vi "security_encrypt.vi"(3 "FORMULA":string, 4 "METHOD":u16(ring) items=["#0_none", "#1_hexa", "#2_hexa_scrambled"], 6 "RAW DATA":string) -> (0 "ENCRYPTED DATA":string)   [LabVIEW 2018, in "db_lib R3.lvlib"]
uses:
  db_lib R3.lvlib
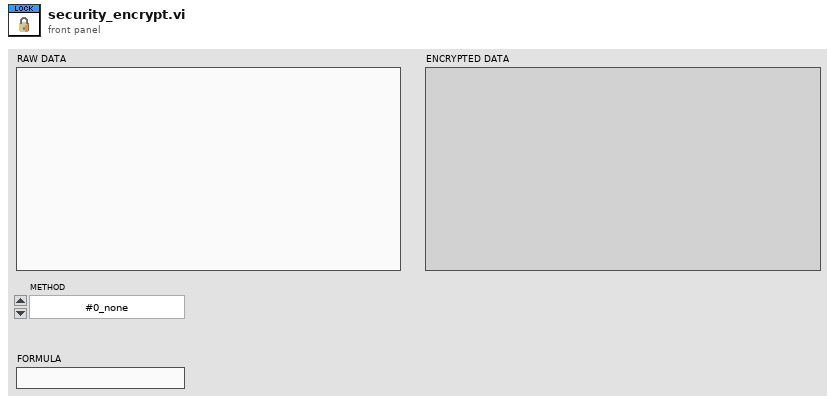
[diagram p1: front panel]
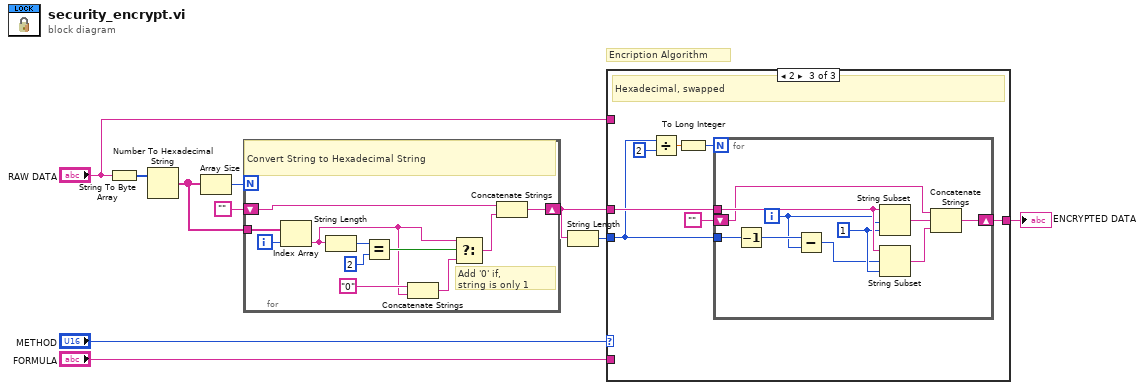
[diagram p0: block diagram]
diagram:
  # "Encription Algorithm"
  n1 = String To Byte Array(string="RAW DATA") -> (unsigned byte array=w10:u8[])
  n2 = Number To Hexadecimal String(2:w10) -> (0:w7:string[])  [unwired: 1 in]
  n3 = Array Size(array=w7) -> (size(s)=w9:i32)
  n4 = for {
    N: w9 -> [_]
    shift-right: [w21] -> w6
    shift-left: "" -> [w20]
    tunnel: w7 -> [w18]
    i -> [w19]
    # "Add '0' if,\nstring is only 1"
    # "Convert String to Hexadecimal String"
    n5 = Index Array(array=w18, index=w19) -> (element=w13:string)
    n6 = String Length(string=w13) -> (length=w17:i32)
    n7 = Equal?(x=w17, y=2) -> (x = y?=w15:bool)
    n8 = Concatenate Strings("0" ("string"), w13) -> (w12:string)
    n9 = Select(t=w13, s=w15, f=w12) -> (s? t:f=w11:string)
    n10 = Concatenate Strings(w20, w11) -> (w21:string)
  }
  n11 = String Length(string=w6) -> (length=w5:i32)
  n12 = case shown="2" "METHOD" {
    tunnel: w6 -> [_ w23 w30]
    tunnel: w5 -> [_ _ w28]
    tunnel: [w22 w23 w24] -> w4
    tunnel: "FORMULA" -> [_ _ _]
    tunnel: "RAW DATA" -> [w22 _ _]
    frame 0, Default {
      # "None"
    }
    frame 1 {
      # "Hexadecimal"
    }
    frame 2 {
      # "Hexadecimal, swapped"
      n13 = Divide(x=w28, y=2) -> (x/y=w27:dbl)
      n14 = To Long Integer(number=w27) -> (32bit integer=w26:i32)
      n15 = for {
        N: w26 -> [_]
        tunnel: w28 -> [w40]
        tunnel: w30 -> [w39]
        shift-right: [w32] -> w24
        shift-left: "" -> [w31]
        i -> [w33]
        w38 = 1 ("length (rest)")
        n16 = Decrement(x=w40) -> (x-1=w34:i32)
        n17 = Subtract(x=w34, y=w33) -> (x-y=w37:i32)
        n18 = String Subset(string=w39, offset (0)=w33, length (rest)=w38) -> (substring=w36:string)
        n19 = String Subset(string=w39, offset (0)=w37, length (rest)=w38) -> (substring=w35:string)
        n20 = Concatenate Strings(w31, w36, w35) -> (w32:string)
      }
    }
  }
  "ENCRYPTED DATA" <- w4
